vi "CheckShot2Shot.vi"(6 "IntensityArray_IN":u8[][](array[numeric]), 11 "ShotArray_IN":T1[](array[typedef])) -> (3 "ShotArray_OUT":T1[](array[typedef]), 4 "IntensityArray_OUT":u8[][](array[numeric]))   [LabVIEW 2022 SP3]
uses:
  ShotCluster.ctl
  move_dir_ud.ctl
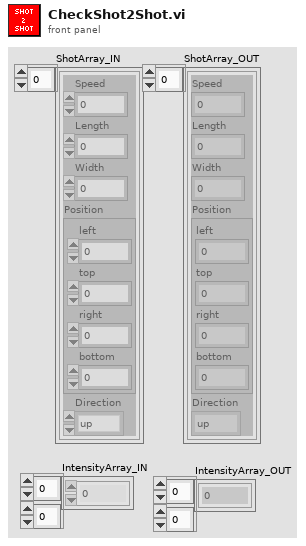
[diagram p1: front panel]
types:
  T1 = typedef "ShotCluster.ctl" = cluster{"Speed":u32, "Length":u32, "Width":u32, "Position":cluster{"left":i16, "top":i16, "right":i16, "bottom":i16}, "Direction":T2}
  T2 = typedef "move_dir_ud.ctl" = enum16{"up", "down"}
  T3 = cluster{"left":i16, "top":i16, "right":i16, "bottom":i16}
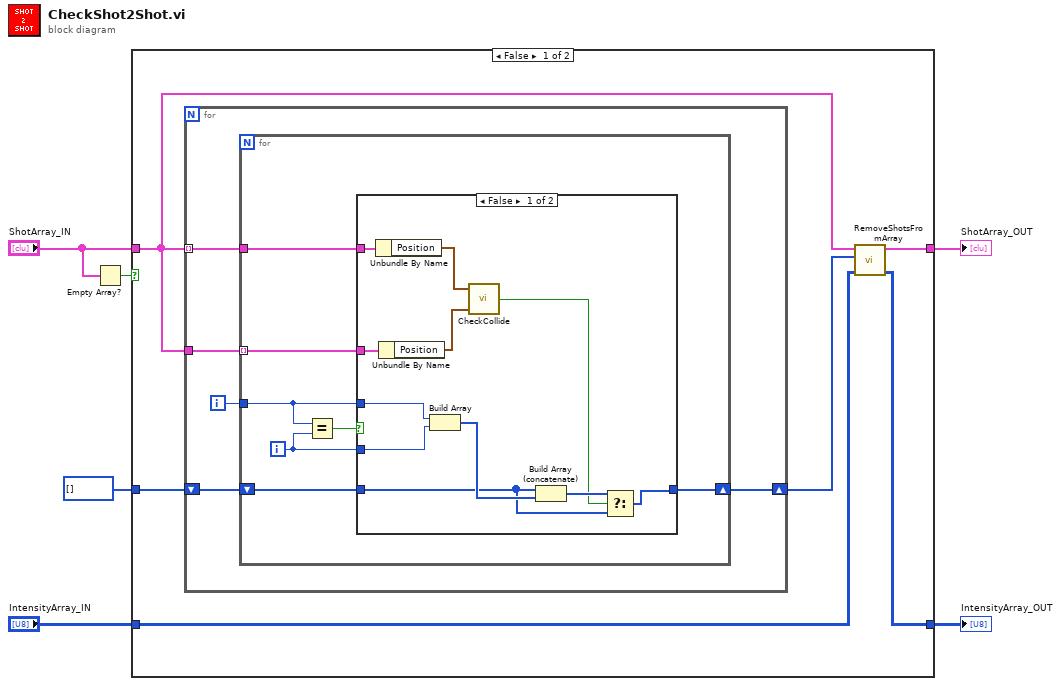
[diagram p0: block diagram]
diagram:
  n1 = Empty Array?(array="ShotArray_IN") -> (empty?=w6:bool)
  n2 = case shown="False" w6 {
    tunnel: "ShotArray_IN" -> [w11 w38]
    tunnel: i32[] [] -> [w12 _]
    tunnel: [w10 w38] -> w3
    tunnel: "IntensityArray_IN" -> [w8 w37]
    tunnel: [w7 w37] -> w1
    frame False {
      n3 = for {
        tunnel: w11 -> [w17] mode=indexing
        tunnel: w11 -> [w16]
        shift-right: [w13] -> w9
        shift-left: w12 -> [w14]
        i -> [w15]
        n4 = for {
          tunnel: w17 -> [w24]
          tunnel: w16 -> [w23] mode=indexing
          tunnel: w15 -> [w21]
          shift-right: [w18] -> w13
          shift-left: w14 -> [w19]
          i -> [w20]
          n5 = Equal?(x=w21, y=w20) -> (x = y?=w22:bool)
          n6 = case shown="False" w22 {
            tunnel: w24 -> [w29 _]
            tunnel: w23 -> [w28 _]
            tunnel: w21 -> [w35 _]
            tunnel: w20 -> [w34 _]
            tunnel: w19 -> [w31 w36]
            tunnel: [w30 w36] -> w18
            frame False {
              n7 = Unbundle By Name(w29) -> ("Position"=w27:T3)
              n8 = Unbundle By Name(w28) -> ("Position"=w26:T3)
              n9 = Build Array(w35, w34) -> (w33:i32[])
              n10 = call "CheckCollide.vi"("Rectangle2"=w26, "Rectangle1"=w27) -> ("Collide"=w25:bool)  [unwired: 3 in]
              n11 = Build Array (concatenate)(w31, w33) -> (w32:i32[])
              n12 = Select(t=w32, s=w25, f=w31) -> (s? t:f=w30:i32[])
            }
            frame True {
            }
          }
        }
      }
      n13 = call "RemoveShotsFromArray.vi"("IntensityArray_IN"=w8, "Indexes"=w9, "ShotArray_IN"=w11) -> ("IntensityArray_OUT"=w7:u8[][], "ShotArray_OUT"=w10:T1[])  [unwired: 7 in]
    }
    frame True {
    }
  }
  "ShotArray_OUT" <- w3
  "IntensityArray_OUT" <- w1
